vi "ex1_3a.vi"() -> ()   [LabVIEW 2017]
uses:
  <vilib>/measure/NI_MABase.lvlib
panel:
  in  "stop":bool
  in  "Sampling parameters":cluster{"Fs":dbl, "Samples":dbl}={"Fs"=2000.0, "Samples"=200.0}
  out "Waveform Graph":waveform(dbl)(graph)
  in  "Phase":dbl
  in  "Amplitude":dbl
  in  "Frequency":dbl
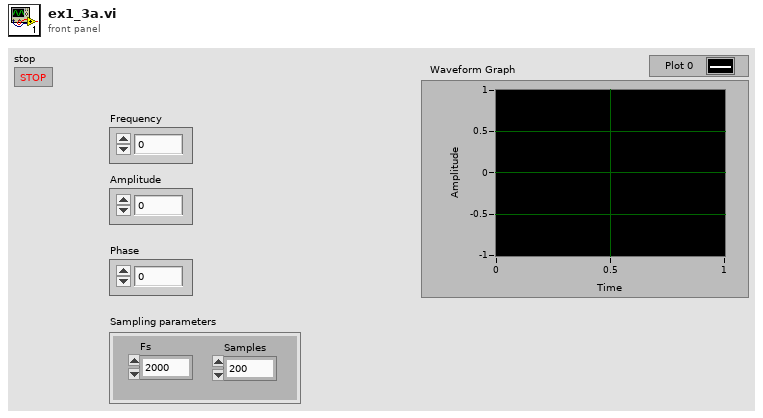
[diagram p1: front panel]
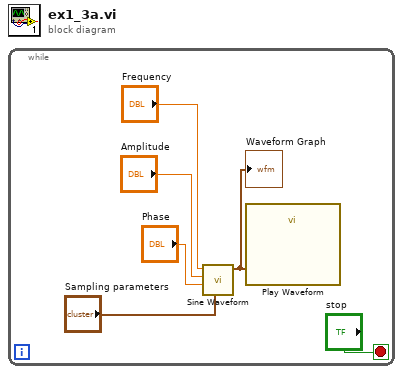
[diagram p0: block diagram]
diagram:
  n1 = while {
    stop <- "stop" stop-if-true
    n2 = call <vilib>:"Sine Waveform.vi"("sampling info"="Sampling parameters", "phase"="Phase", "amplitude"="Amplitude", "frequency"="Frequency") -> ("signal out"=w2:waveform(dbl))  [unwired: 6 in, 1 out]
    "Waveform Graph" <- w2
    n3 = call "Play Waveform"("Data"=w2) -> ()  [unwired: 18 in, 1 out]
  }
